vi "Track Dropped Frames_atw1.vi"(6 "NumLost":u32[](array[numeric]), 7 "BuffNum":u32[](array[numeric]), 8 "Curr Buffer":u32, 9 "Prev Lost":u32, 10 "Prev Buffer":u32) -> (3 "New Lost":u32, 4 "NewNumLost":u32[](array[numeric]), 5 "NewBuffNum":u32[](array[numeric]))   [LabVIEW 2013]
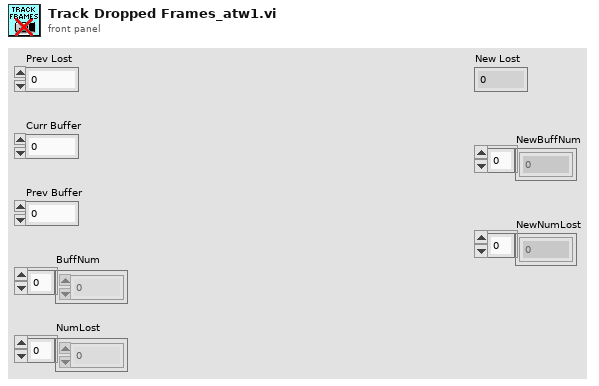
[diagram p1: front panel]
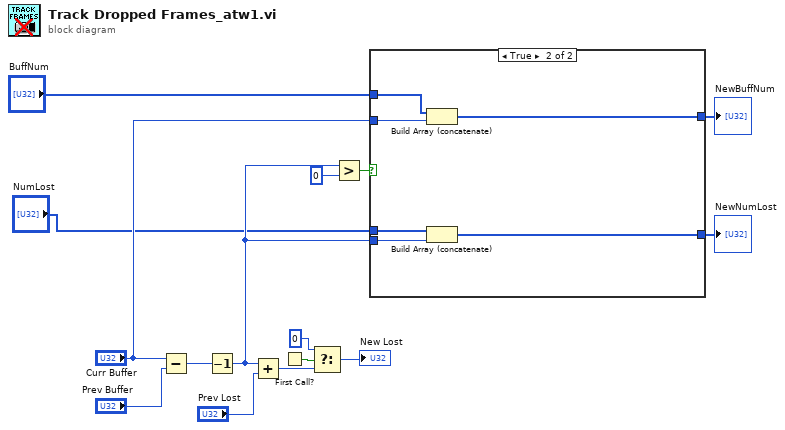
[diagram p0: block diagram]
diagram:
  n1 = Subtract(x="Curr Buffer", y="Prev Buffer") -> (x-y=w15:u32)
  n2 = Decrement(x=w15) -> (x-1=w5:u32)
  n3 = Add(x=w5, y="Prev Lost") -> (x+y=w14:u32)
  n4 = First Call?() -> (First Call?: T/F=w12:bool)
  n5 = Select(t=u32 0, s=w12, f=w14) -> (s? t:f=→"New Lost":u32)
  n6 = Greater?(x=w5, y=u32 0) -> (0:w8:bool)
  n7 = case shown="True" w8 {
    tunnel: "Curr Buffer" -> [_ w23]
    tunnel: w5 -> [_ w22]
    tunnel: "NumLost" -> [w16 w21]
    tunnel: "BuffNum" -> [w17 w20]
    tunnel: [w17 w19] -> w2
    tunnel: [w16 w18] -> w1
    frame False {
    }
    frame True {
      n8 = Build Array (concatenate)(w20, w23) -> (w19:u32[])
      n9 = Build Array (concatenate)(w21, w22) -> (w18:u32[])
    }
  }
  "NewBuffNum" <- w2
  "NewNumLost" <- w1
